vi "PPSU Ramp FGV.vi"(7 "Write/Read":T1=enum."Read", 8 "error in":errorcluster, 10 "PPSU update Voltage(W)":dbl) -> (0 "error out":errorcluster, 2 "PPSU update Voltage (R)":dbl)   [LabVIEW 2022 SP3]
uses:
  Controls/FGV Read write.ctl
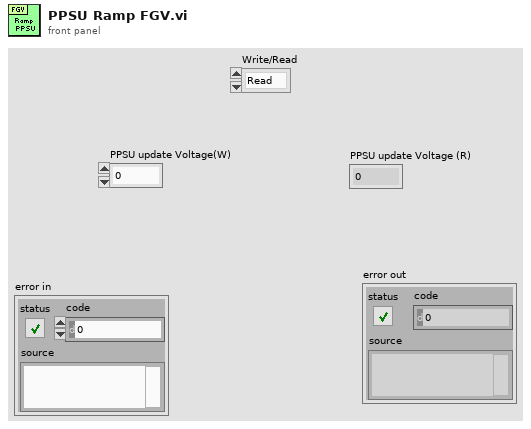
[diagram p1: front panel]
types:
  T1 = typedef "FGV Read write.ctl" = enum16{"Write", "Read"}
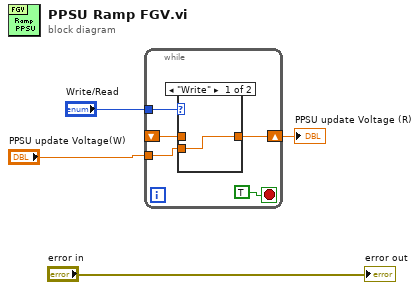
[diagram p0: block diagram]
diagram:
  n1 = while {
    tunnel: "Write/Read" -> [w8]
    shift-right: [w7] -> w1
    shift-left: _ -> [w6]
    tunnel: "PPSU update Voltage(W)" -> [w5]
    stop <- TRUE stop-if-true
    n2 = case shown="\"Write\"" w8 {
      tunnel: [w10 w11] -> w7
      tunnel: w6 -> [_ w11]
      tunnel: w5 -> [w10 _]
      frame "Write" {
      }
      frame "Read" {
      }
    }
  }
  "PPSU update Voltage (R)" <- w1
  "error out" <- "error in"
